vi "BLM_MotorDisabledWarning.vi"(5 "BLM Status":bool[](array[boolean]), 6 "BLM Alarm Code":bool[](array[boolean]), 7 "Instrument Address":refnum<visa-resource-name>) -> (1 "Which Button?":T1(ring)=enum."Center Button", 2 "Ignore Alarms":bool, 3 "Instrument Address Out":refnum<visa-resource-name>)   [LabVIEW 2019]
panel:
  # "Alarm code:\nHex Value for BLu drive\n0001 Position Limit\n0002 CCW Limit\n0004 CW Limit\n0008 Over Temp\n0010 Excess Regen* \n0020 Over Voltage\n0040 Under Voltage* \n0080 Over Current\n0100 Bad Hall Sensor \n0200 Bad Encoder \n0400 Comm Error\n0800 Bad Flash\n1000 Wizard Failed \n2000 Current Foldback \n4000 Blank Q Segment\n8000 No Move \n* BLuAC drives only\nNOTE: Items in bold italic represent \nDrive Faults, \nwhich automatically disable the motor."
  # "SC command - Response Details:\nHex Value Status Code bit definition\n0001 Motor Enabled (Motor Disabled if this bit = 0)\n0002 Sampling (for Quick Tuner)\n0004 Drive Fault (check Alarm Code)\n0008 In Position (motor is in position)\n0010 Moving (motor is moving)\n0020 Jogging (currently in jog mode)\n0040 Stopping (in the process of stopping from a stop command)\n0080 Waiting (for an input)\n0100 Saving (parameter data is being saved)\n0200 Alarm present (check Alarm Code)\n0400 Homing (executing an SH command)\n0800 Wait Time (executing a WT command)\n1000 Wizard running (Timing Wizard is running)\n2000 Checking encoder (Timing Wizard is running)\n4000 Q Program is running\n8000 Initializing (happens at power up)"
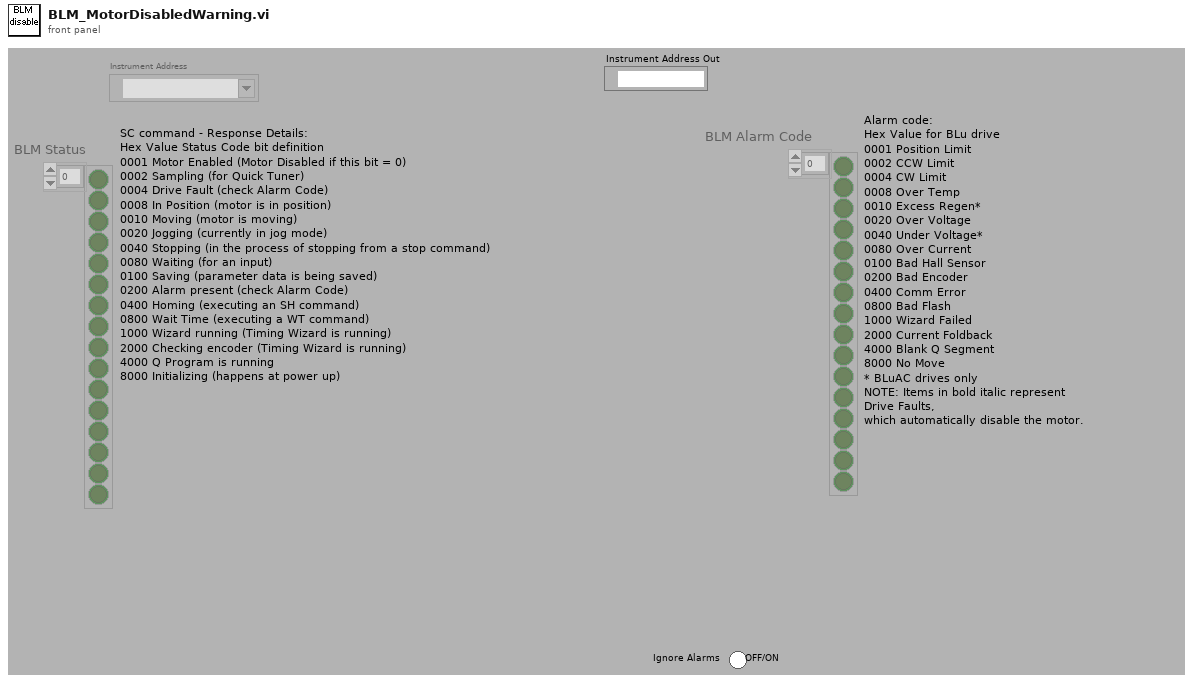
[diagram p1: front panel]
types:
  T1 = enum16{"Left Button", "Center Button", "Right Button", "Window Close"}
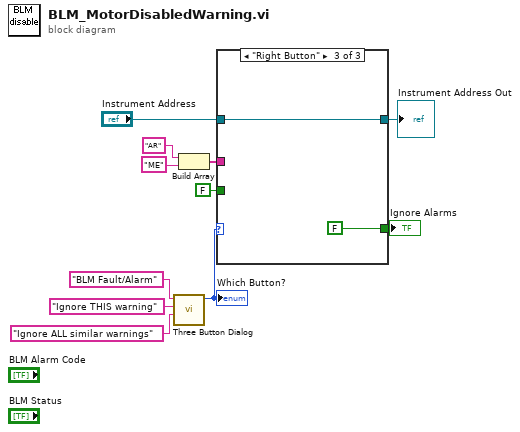
[diagram p0: block diagram]
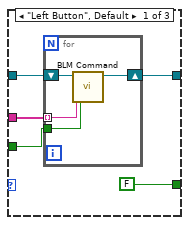
[diagram p2: hidden frame]
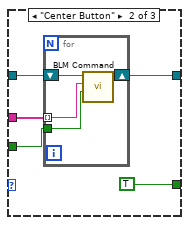
[diagram p3: hidden frame]
diagram:
  n1 = call <vilib>:"Three Button Dialog.vi"("Center Button Text (\"No\")"="Ignore ALL similar warnings" ("Center Button Text (\"No\")"), "Left Button Text (\"Yes\")"="Ignore THIS warning" ("T button name (\"OK\")"), "message"="BLM Fault/Alarm") -> ("Which Button?"=w8:T1)  [unwired: 8 in]
  "Which Button?" <- w8
  n2 = Build Array("AR" ("Command"), "ME" ("Command")) -> (w3:string[])
  n3 = case shown="\"Right Button\"" w8 {
    tunnel: "Instrument Address" -> [w16 w25 w30]
    tunnel: w3 -> [w15 w24 _]
    tunnel: FALSE ("Read Echo?") -> [w14 w23 _]
    tunnel: [FALSE ("Read Echo?") TRUE ("Read Echo?") FALSE ("Read Echo?")] -> w2
    tunnel: [w12 w21 w30] -> w1
    frame "Left Button", Default {
      n4 = for {
        tunnel: w15 -> [w19] mode=indexing
        tunnel: w14 -> [w18]
        shift-right: [w17] -> w12
        shift-left: w16 -> [w20]
        n5 = call "BLM Command.vi"("Read Echo?"=w18, "Command"=w19, "Port Address"=w20) -> ("Port Address Out"=w17:refnum<visa-resource-name>)  [unwired: 3 in, 4 out]
      }
    }
    frame "Center Button" {
      n6 = for {
        tunnel: w24 -> [w28] mode=indexing
        tunnel: w23 -> [w27]
        shift-right: [w26] -> w21
        shift-left: w25 -> [w29]
        n7 = call "BLM Command.vi"("Read Echo?"=w27, "Command"=w28, "Port Address"=w29) -> ("Port Address Out"=w26:refnum<visa-resource-name>)  [unwired: 3 in, 4 out]
      }
    }
    frame "Right Button" {
    }
  }
  "Ignore Alarms" <- w2
  "Instrument Address Out" <- w1
